vi "Init.vi"(8 "error in (no error)":errorcluster, 11 "Serial in":refnum<class "Serial.lvclass">) -> (0 "error out":errorcluster, 3 "Serial out":refnum<class "Serial.lvclass">)   [LabVIEW 2021, in "Serial.lvclass"]
uses:
  Serial.lvclass
  C:/Users/enric/Desktop/mpb/Type Defs/Serial - Settings.ctl
  Serial.lvclass/Serial.ctl
  <vilib>/Instr/_visa.llb/VISA Configure Serial Port (Instr).vi
panel:
  in  "Serial Settings":T1={"baud rate"=115200, "data bits"=8, "parity"=enum."None", "stop bits"=10, "flow control"=0} {"flow control" items=["None"=0, "XON/XOFF"=1, "RTS/CTS"=2, "DTR/DSR"=4]; "stop bits" items=["1.0"=10, "1.5"=15, "2.0"=20]; "data bits" min=5 max=8 step=1}
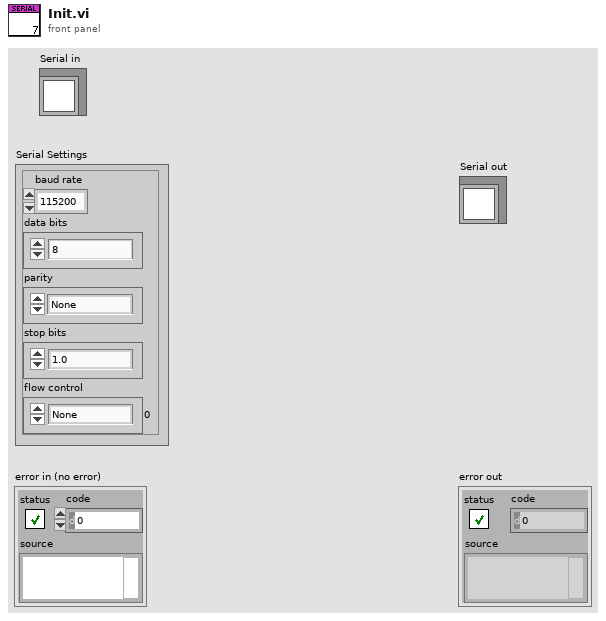
[diagram p1: front panel]
types:
  T1 = typedef "Serial - Settings.ctl" = cluster{"baud rate":u32, "data bits":u16, "parity":enum16{"None", "Odd", "Even", "Mark", "Space"}, "stop bits":u16, "flow control":u16}
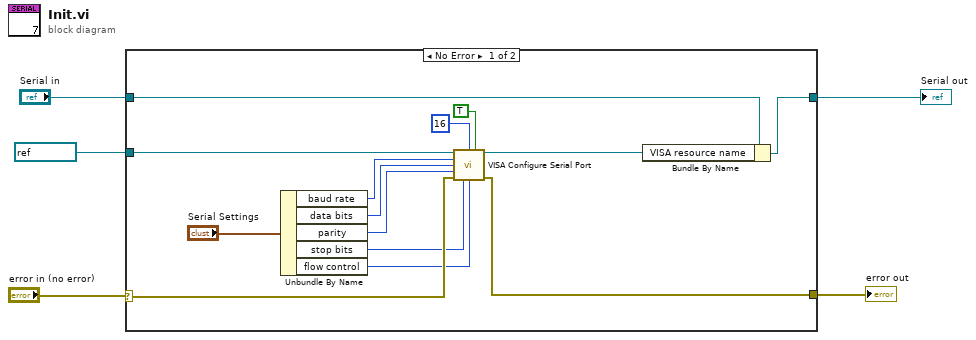
[diagram p0: block diagram]
diagram:
  n1 = case shown="No Error" "error in (no error)" {
    selector: "error in (no error)" -> [w19 w21]
    tunnel: [w6 w21] -> w4
    tunnel: "Serial in" -> [w9 w20]
    tunnel: [w8 w20] -> w2
    tunnel: refnum<visa-resource-name> "COM8" ("VISA resource name") -> [w10 _]
    frame No Error {
      n2 = Unbundle By Name("Serial Settings") -> ("baud rate"=w17:u32, "data bits"=w16:u16, "parity"=w15:enum16{"None", "Odd", "Even", "Mark", "Space"}, "stop bits"=w12:u16, "flow control"=w11:u16)
      n3 = call-poly "VISA Configure Serial Port"("VISA resource name"=w10, "termination char\n(0xA = '\\n' = LF)"=u8 16 ("termination char\n(0xA = '\\n' = LF)"), "Enable Termination\nChar (T)"=TRUE ("Enable Termination\nChar (T)"), "baud rate (9600)"=w17, "data bits (8)"=w16, "parity (0:none)"=w15, "error in (no error)"=w19, "stop bits (10: 1 bit)"=w12, "flow control (0:none)"=w11) -> ("VISA resource name out"=w7:refnum<visa-resource-name>, "error out"=w6:errorcluster)  [unwired: 5 in]
      n4 = Bundle By Name(cluster=w9, "VISA resource name"=w7) -> (w8:refnum<class "Serial.lvclass">)
    }
    frame Error {
    }
  }
  "error out" <- w4
  "Serial out" <- w2
